vi "Method.vi"(4 "Value B":refnum<class "Abs_Numeric.lvclass">, 5 "Value A":refnum<class "Abs_Extended Float.lvclass">) -> (1 "Result":refnum<class "Abs_Boolean.lvclass">)   [LabVIEW 2021, in "Greater_EXT.lvclass"]
uses:
  Greater_EXT.lvclass
  Abs_Types/Extended Float/Abs_Extended Float.lvclass
  Abs_Types/Boolean/Abs_Boolean.lvclass
  Abs_Types/Numeric/Abs_Numeric.lvclass
  C:/TSA/LV_Abstract/Source/Functions/Support/Compare/Two Term/EXT/AbsComp_Two Term_EXT.lvclass
  C:/Program Files (x86)/National Instruments/LabVIEW 2021/vi.lib/TSA/Abstract Data Classes/Abs_Types/Boolean/Abs_Boolean.lvclass
  Support/Compare/Two Term/EXT/AbsComp_Two Term_EXT.lvclass/AbsComp_Two Term_EXT.ctl
  Support/Compare/Two Term/EXT/Properties/Write Numeric A.vi
  Support/Compare/Two Term/EXT/Properties/Write Numeric B.vi
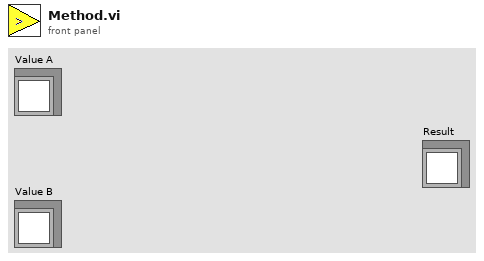
[diagram p1: front panel]
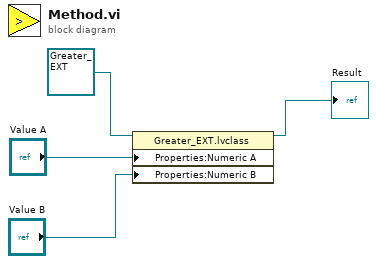
[diagram p0: block diagram]
diagram:
  n1 = property class="Greater_EXT.lvclass"(reference=refnum<class "Greater_EXT.lvclass"> refnum ("Greater 0_U64.lvclass"), "Properties:Numeric A"="Value A", "Properties:Numeric B"="Value B") -> (reference out=→"Result":refnum<class "Greater_EXT.lvclass">)  [unwired: 1 in, 1 out]
